vi "Read String.vi"(2 "Network Path":string, 5 "Tag Name":string) -> (1 "String":string)   [LabVIEW 2020]
uses:
  <vilib>/ethernetip/ethernetip.llb/EthernetIP Tag Read STRING.vi
  <vilib>/ethernetip/ethernetip.lvlib
panel:
  out "error out":errorcluster
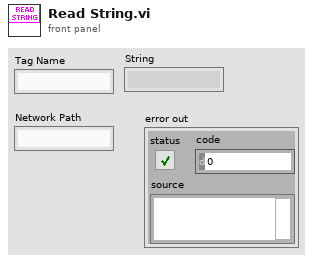
[diagram p1: front panel]
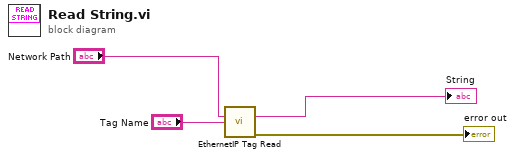
[diagram p0: block diagram]
diagram:
  n1 = call-poly <vilib>:"EthernetIP Tag Read.vi"("Network Path"="Network Path", "Tag Name"="Tag Name") -> ("Data"=→"String":string, "error out"=→"error out":errorcluster)  [unwired: 2 in, 10 out]
